vi "GE 5565PIORC.Pointer.Dispose.vi"(8 "error in (no error)":errorcluster, 11 "pointer":u64 format="%08x") -> (0 "error out":errorcluster)   [LabVIEW 2020, in "GE 5565PIORC.lvclass"]
doc: "Deallocates the memory associated with <b>pointer</b>, previously allocated by Pointer.New."
uses:
  GE 5565PIORC.lvclass
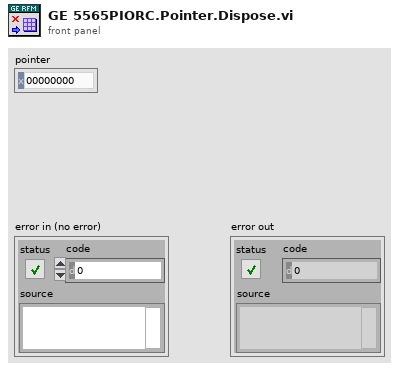
[diagram p1: front panel]
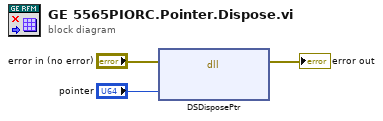
[diagram p0: block diagram]
diagram:
  n1 = dll-call lib="LabVIEW" fn="DSDisposePtr"(error in="error in (no error)", "pointer"="pointer") -> (error out=→"error out":errorcluster)  [unwired: 4 in, 1 out]
